vi "practica 2.vi"() -> ()   [LabVIEW 2014]
panel:
  out "Waveform Chart":dynamicdata(graph)
  in  "stop (F) 2":bool caption="stop (F)"
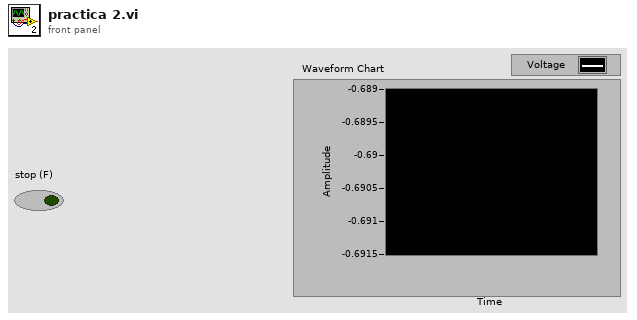
[diagram p1: front panel]
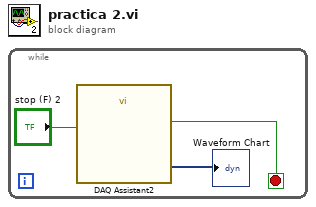
[diagram p0: block diagram]
diagram:
  n1 = while {
    stop <- w2 stop-if-true
    n2 = call "DAQ Assistant2"("stop (F)"="stop (F) 2") -> ("data"=→"Waveform Chart":dynamicdata, "stopped"=w2:bool)  [unwired: 15 in, 2 out]
  }
